vi "SP Append Group Data Fields.vi"(10 "S Parameter Results":T1={"Measurement Cycles"=0, "Sxx Data"=[], "S Parameter Test Parameters"={"Stimulus"={"Use Instrument Settings"=FALSE, "Blank Frequencies"=FALSE, "Sweep Type"=enum."Linear", "Sweep"={"Fstart"=500.0, "Fstop"=1500.0, "Units"=enum."MHz", "Points"=2}, "Power (dBm)"=999.0, "IFBW (Hz)"=-1.0, "Sweep Time (s)"=-1.0, "Calibration"={"State"=FALSE, "String"=""}}, "Measurement"={"Auto Select"=TRUE, "Data Source"=enum."VNA", "Ports"=2, "Parameters"=[]}, "De-Embed"={"De-Embed"=FALSE, "Adapters"=[]}, "Display"={"Lock Control"=FALSE, "Retain Settings"=TRUE, "Formatted Data"=FALSE, "Plot Orientation"=enum."Single", "Plot Controls"=[{"Trace Orientation"=enum."Overlay", "Frequency"={"Change Frequency"=FALSE, "Start"=500.0, "Stop"=1500.0, "Units"=enum."MHz"}, "Markers"=[], "Traces"=[]}, {"Trace Orientation"=enum."Overlay", "Frequency"={"Change Frequency"=FALSE, "Start"=500.0, "Stop"=1500.0, "Units"=enum."MHz"}, "Markers"=[], "Traces"=[]}, {"Trace Orientation"=enum."Overlay", "Frequency"={"Change Frequency"=FALSE, "Start"=500.0, "Stop"=1500.0, "Units"=enum."MHz"}, "Markers"=[], "Traces"=[]}, {"Trace Orientation"=enum."Overlay", "Frequency"={"Change Frequency"=FALSE, "Start"=500.0, "Stop"=1500.0, "Units"=enum."MHz"}, "Markers"=[], "Traces"=[]}]}, "Limits"=[], "Filter Limits"=[]}, "Instrument Used"={"ixInstrument"=0, "sxInstrumentId"="", "sDriverId"="", "sDriverType"="", "sSerialNumber"="", "tLastCalibration"=timestamp(0 s since 1904-01-01), "tCalibrationDue"=timestamp(0 s since 1904-01-01), "sConfiguration"=""}} {"S Parameter Test Parameters"."Filter Limits"."Parameter"."Stimulus Port" min=1 step=1; "S Parameter Test Parameters"."Filter Limits"."Parameter"."Response Port" min=1 step=1; "S Parameter Test Parameters"."Filter Limits"."Passband"."Bandwidth Attn" format="%.3g"; "S Parameter Test Parameters"."Filter Limits"."Passband"."Stop/Span" format="%.3g"; "S Parameter Test Parameters"."Filter Limits"."Passband"."Start/Center" format="%.3g"; "S Parameter Test Parameters"."Measurement"."Parameters"."Channel" min=0 max=32 step=1; "S Parameter Test Parameters"."Measurement"."Parameters"."Parameter"."Stimulus Port" min=1 step=1; "S Parameter Test Parameters"."Measurement"."Parameters"."Parameter"."Response Port" min=1 step=1; "S Parameter Test Parameters"."Limits"."Parameter"."Stimulus Port" min=1 step=1; "S Parameter Test Parameters"."Limits"."Parameter"."Response Port" min=1 step=1; "S Parameter Test Parameters"."Stimulus"."Sweep Time (s)" format="%.3g"; "S Parameter Test Parameters"."Display"."Plot Controls"."Traces"."Reference" format="%#.2g"; "S Parameter Test Parameters"."Display"."Plot Controls"."Traces"."Scale" min=0.001 step=1.0 format="%#.2g"; "S Parameter Test Parameters"."Display"."Plot Controls"."Traces"."Position" min=0.0 max=10.0; "S Parameter Test Parameters"."Display"."Plot Controls"."Frequency"."Stop" format="%.3g"; "S Parameter Test Parameters"."Display"."Plot Controls"."Frequency"."Start" format="%.3g"}, 11 "Fields In":T34[](array[typedef])) -> (3 "Fields Out":T34[](array[typedef]))   [LabVIEW 2011]
uses:
  server/database/Fields/Field Record.ctl
  server/database/Fields/Field DataTypes.ctl
  server/database/Fields/Field NextItem.ctl
  TypeDefs/SP Results.ctl
  TypeDefs/SP Test Parameters.ctl
  TypeDefs/SP Stimulus Parameters.ctl
  TypeDefs/SP Frequency Units.ctl
  TypeDefs/SP Calibration State.ctl
  TypeDefs/SP Measurement.ctl
  TypeDefs/SP Parameters.ctl
  TypeDefs/SP Parameter.ctl
  TypeDefs/SP De-Embed.ctl
  TypeDefs/SP Adapter.ctl
  TypeDefs/SP Data.ctl
  TypeDefs/SP Display Parameters.ctl
  TypeDefs/SP Display Plot Controls Cluster.ctl
  TypeDefs/SP Marker Cluster.ctl
  TypeDefs/SP Marker Type.ctl
  TypeDefs/SP Display Trace Controls.ctl
  TypeDefs/SP Display Format.ctl
  TypeDefs/SP Display Data.ctl
  TypeDefs/SP Limit.ctl
  TypeDefs/SP Format.ctl
  TypeDefs/SP Limit Type.ctl
  TypeDefs/SP Limit Point.ctl
  Test Referential Limit.ctl
  TypeDefs/SP Filter.ctl
  TypeDefs/SP Filter Type.ctl
  TypeDefs/SP Filter Passband.ctl
  TypeDefs/SP Frequency Format.ctl
  TypeDefs/SP Filter Ripple.ctl
  TypeDefs/SP Attenuation Point.ctl
  TypeDefs/SP Attenuation Type.ctl
  TypeDefs/SP Skirt Rejection Point.ctl
  TypeDefs/SP Relative Loss.ctl
  server/database/Stations/Instruments/Instrument Record.ctl
panel:
  # "Div"
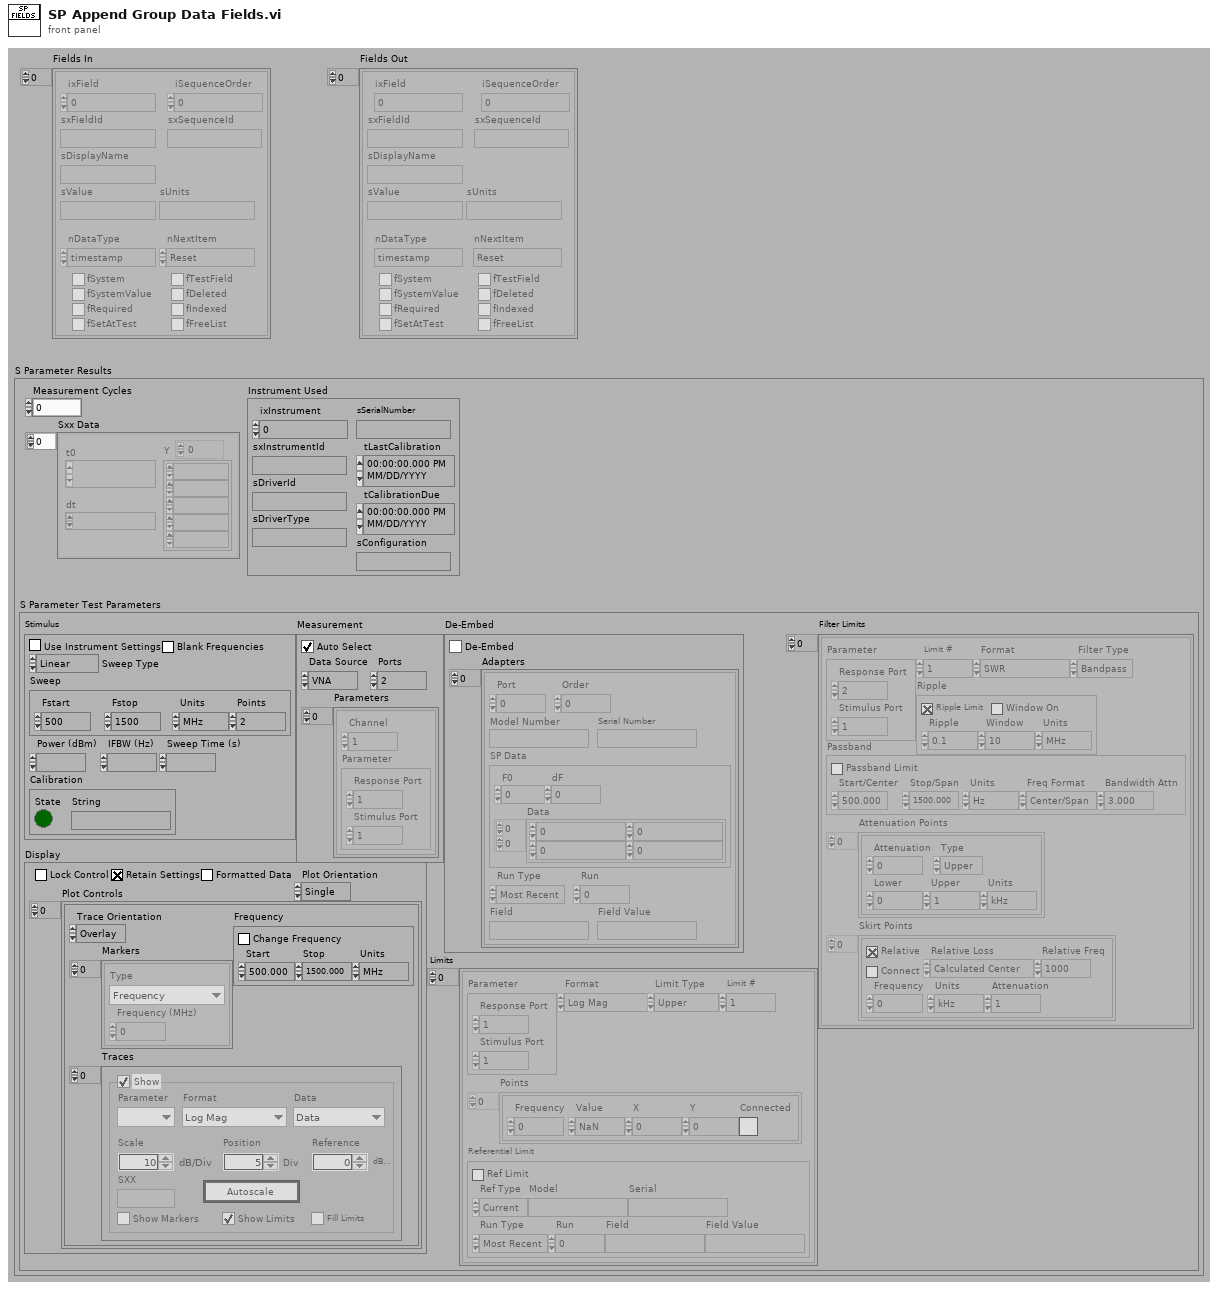
[diagram p1: front panel]
types:
  T1 = typedef "SP Results.ctl" = cluster{"Measurement Cycles":i32, "Sxx Data":waveform(dbl)[], "S Parameter Test Parameters":T2, "Instrument Used":T33}
  T2 = typedef "SP Test Parameters.ctl" = cluster{"Stimulus":T3, "Measurement":T6, "De-Embed":T9, "Display":T12, "Limits":T19[], "Filter Limits":T24[]}
  T3 = typedef "SP Stimulus Parameters.ctl" = cluster{"Use Instrument Settings":bool, "Blank Frequencies":bool, "Sweep Type":enum32{"Linear", "Logarithmic", "List", "Power", "CW"}, "Sweep":cluster{"Fstart":dbl, "Fstop":dbl, "Units":T4, "Points":i32}, "Power (dBm)":dbl, "IFBW (Hz)":dbl, "Sweep Time (s)":dbl, "Calibration":T5}
  T4 = typedef "SP Frequency Units.ctl" = enum16{"Hz", "kHz", "MHz", "GHz", "Points"}
  T5 = typedef "SP Calibration State.ctl" = cluster{"State":bool, "String":string}
  T6 = typedef "SP Measurement.ctl" = cluster{"Auto Select":bool, "Data Source":enum16{"VNA", "Data File"}, "Ports":i8, "Parameters":T7[]}
  T7 = typedef "SP Parameters.ctl" = cluster{"Channel":i8, "Parameter":T8}
  T8 = typedef "SP Parameter.ctl" = cluster{"Stimulus Port":i8, "Response Port":i8}
  T9 = typedef "SP De-Embed.ctl" = cluster{"De-Embed":bool, "Adapters":T10[]}
  T10 = typedef "SP Adapter.ctl" = cluster{"Port":i8, "Order":i8, "Model Number":string, "Serial Number":string, "SP Data":T11, "Run Type":enum16{"Most Recent", "Run #", "Match Field"}, "Run":i32, "Field":string, "Field Value":string}
  T11 = typedef "SP Data.ctl" = cluster{"F0":dbl, "dF":dbl, "Data":cdb[][]}
  T12 = typedef "SP Display Parameters.ctl" = cluster{"Lock Control":bool, "Retain Settings":bool, "Formatted Data":bool, "Plot Orientation":enum32{"Single", "Dual", "Quad"}, "Plot Controls":T13[]}
  T13 = typedef "SP Display Plot Controls Cluster.ctl" = cluster{"Trace Orientation":enum32{"Overlay", "Split"}, "Frequency":cluster{"Change Frequency":bool, "Start":dbl, "Stop":dbl, "Units":T4}, "Markers":T14[], "Traces":T16[]}
  T14 = typedef "SP Marker Cluster.ctl" = cluster{"Type":T15, "Frequency (MHz)":dbl}
  T15 = typedef "SP Marker Type.ctl" = enum16{"Frequency", "Trace Maximum", "Trace Minimum", "Limit Maximum", "Limit Minimum"}
  T16 = typedef "SP Display Trace Controls.ctl" = cluster{"Trace On":bool, "Measure":i32, "Format":T17, "Autoscale":bool, "Reference":dbl, "\nRefUnit":string, "Position":dbl, "Scale":dbl, "ScaleUnit":string, "LimitOn":bool, "LimitFill":bool, "Display Data":T18, "Show Markers":bool, "SXX":string}
  T17 = typedef "SP Display Format.ctl" = i32
  T18 = typedef "SP Display Data.ctl" = u16
  T19 = typedef "SP Limit.ctl" = cluster{"Parameter":T8, "Format":T20, "Limit Type":T21, "Points":T22[], "Referential Limit":T23, "Limit #":i8}
  T20 = typedef "SP Format.ctl" = enum16{"Log Mag", "Lin Mag", "SWR", "Phase", "Expanded Phase", "Delay", "Insertion Loss", "Isolation", "Return Loss"}
  T21 = typedef "SP Limit Type.ctl" = enum16{"Upper", "Lower", "Delta", "Filter", "Referential"}
  T22 = typedef "SP Limit Point.ctl" = cluster{"Frequency":dbl, "Value":dbl, "X":dbl, "Y":dbl, "Connected":bool}
  T23 = typedef "Test Referential Limit.ctl" = cluster{"Ref Limit":bool, "Ref Type":enum16{"Current", "Specify"}, "Model":string, "Serial":string, "Run Type":enum16{"Most Recent", "Run #", "Match Field"}, "Run":i32, "Field":string, "Field Value":string}
  T24 = typedef "SP Filter.ctl" = cluster{"Limit #":i8, "Parameter":T8, "Format":T20, "Filter Type":T25, "Passband":T26, "Ripple":T28, "Attenuation Points":T29[], "Skirt Points":T31[]}
  T25 = typedef "SP Filter Type.ctl" = enum16{"Lowpass", "Highpass", "Bandpass", "Bandstop"}
  T26 = typedef "SP Filter Passband.ctl" = cluster{"Start/Center":dbl, "Stop/Span":dbl, "Units":T4, "Freq Format":T27, "Bandwidth Attn":dbl, "Passband Limit":bool}
  T27 = typedef "SP Frequency Format.ctl" = enum16{"Start/Stop", "Center/Span"}
  T28 = typedef "SP Filter Ripple.ctl" = cluster{"Ripple Limit":bool, "Window On":bool, "Ripple":dbl, "Window":dbl, "Units":T4}
  T29 = typedef "SP Attenuation Point.ctl" = cluster{"Attenuation":dbl, "Type":T30, "Lower":dbl, "Upper":dbl, "Units":T4}
  T30 = typedef "SP Attenuation Type.ctl" = enum16{"Center", "Lower", "Upper"}
  T31 = typedef "SP Skirt Rejection Point.ctl" = cluster{"Relative":bool, "Connect":bool, "Frequency":dbl, "Units":T4, "Attenuation":dbl, "Relative Loss":T32, "Relative Freq":dbl}
  T32 = typedef "SP Relative Loss.ctl" = enum16{"Calculated Center", "Passband Minimum", "Passband Maximum", "Passband Average", "Frequency"}
  T33 = typedef "Instrument Record.ctl" = cluster{"ixInstrument":i32, "sxInstrumentId":string, "sDriverId":string, "sDriverType":string, "sSerialNumber":string, "tLastCalibration":timestamp, "tCalibrationDue":timestamp, "sConfiguration":string}
  T34 = typedef "Field Record.ctl" = cluster{"ixField":i32, "iSequenceOrder":i32, "sxFieldId":string, "sxSequenceId":string, "sDisplayName":string, "sValue":string, "sUnits":string, "nDataType":T35, "nNextItem":T36, "fSystem":bool, "fSystemValue":bool, "fRequired":bool, "fSetAtTest":bool, "fTestField":bool, "fDeleted":bool, "fIndexed":bool, "fFreeList":bool}
  T35 = typedef "Field DataTypes.ctl" = enum32{"text", "numeric", "list", "timestamp", "boolean"}
  T36 = typedef "Field NextItem.ctl" = enum32{"Reset", "Retain", "Auto-Increment"}
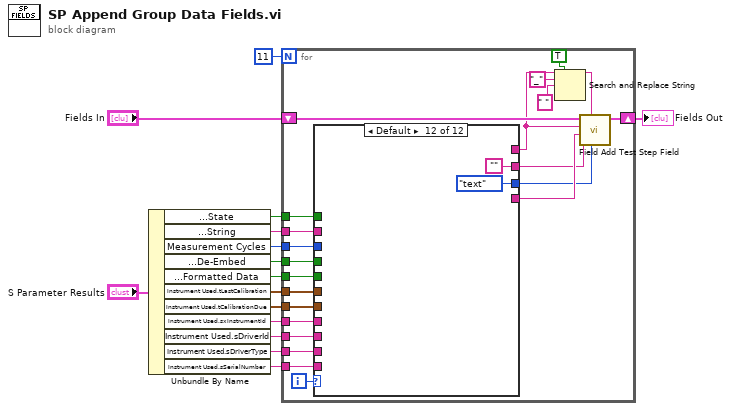
[diagram p0: block diagram]
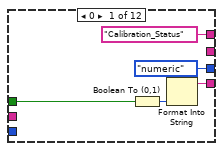
[diagram p2: hidden frame]
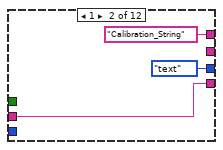
[diagram p3: hidden frame]
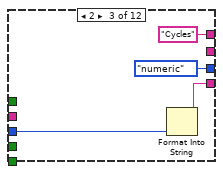
[diagram p4: hidden frame]
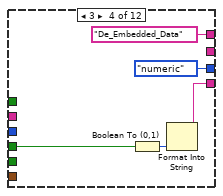
[diagram p5: hidden frame]
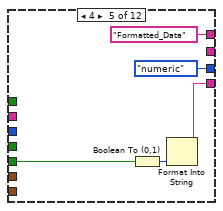
[diagram p6: hidden frame]
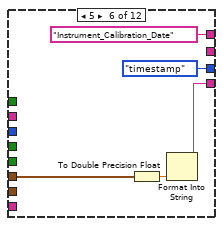
[diagram p7: hidden frame]
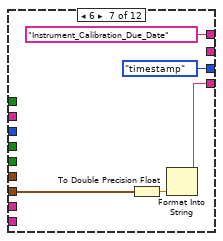
[diagram p8: hidden frame]
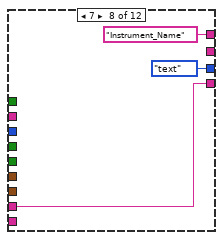
[diagram p9: hidden frame]
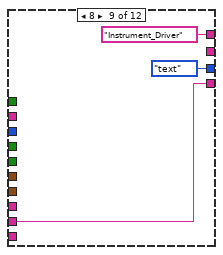
[diagram p10: hidden frame]
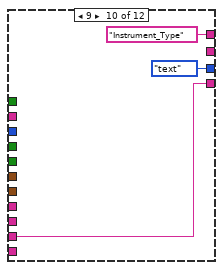
[diagram p11: hidden frame]
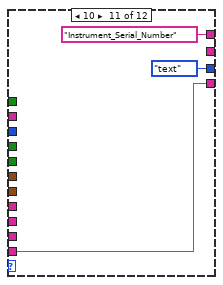
[diagram p12: hidden frame]
diagram:
  n1 = Unbundle By Name("S Parameter Results") -> ("S Parameter Test Parameters.Stimulus.Calibration.State"=w11:bool, "S Parameter Test Parameters.Stimulus.Calibration.String"=w10:string, "Measurement Cycles"=w9:i32, "S Parameter Test Parameters.De-Embed.De-Embed"=w8:bool, "S Parameter Test Parameters.Display.Formatted Data"=w7:bool, "Instrument Used.tLastCalibration"=w6:timestamp, "Instrument Used.tCalibrationDue"=w5:timestamp, "Instrument Used.sxInstrumentId"=w4:string, "Instrument Used.sDriverId"=w3:string, "Instrument Used.sDriverType"=w2:string, "Instrument Used.sSerialNumber"=w1:string)
  n2 = for {
    N: 11 -> [_]
    tunnel: w7 -> [w36]
    tunnel: w8 -> [w35]
    tunnel: w9 -> [w34]
    tunnel: w10 -> [w33]
    tunnel: w11 -> [w32]
    shift-right: [w30] -> w14
    shift-left: "Fields In" -> [w31]
    tunnel: w6 -> [w26]
    tunnel: w5 -> [w25]
    tunnel: w4 -> [w24]
    tunnel: w3 -> [w23]
    tunnel: w2 -> [w22]
    tunnel: w1 -> [w21]
    i -> [w37]
    n3 = case shown="Default" w37 {
      tunnel: w36 -> [_ _ _ _ w56 _ _ _ _ _ _ _]
      tunnel: w35 -> [_ _ _ w51 _ _ _ _ _ _ _ _]
      tunnel: w34 -> [_ _ w47 _ _ _ _ _ _ _ _ _]
      tunnel: w33 -> [_ w43 _ _ _ _ _ _ _ _ _ _]
      tunnel: w32 -> [w39 _ _ _ _ _ _ _ _ _ _ _]
      tunnel: ["Calibration_Status" ("Field_ID") "Calibration_String" ("Field_ID") "Cycles" ("Field_ID") "De_Embedded_Data" ("Field_ID") "Formatted_Data" ("Field_ID") "Instrument_Calibration_Date" ("Field_ID") "Instrument_Calibration_Due_Date" ("Field_ID") "Instrument_Name" ("Field_ID") "Instrument_Driver" ("Field_ID") "Instrument_Type" ("Field_ID") "Instrument_Serial_Number" ("Field_ID") _] -> w16
      tunnel: [Field_DataTypes."numeric" ("Data Type") Field_DataTypes."text" ("Data Type") Field_DataTypes."numeric" ("Data Type") Field_DataTypes."numeric" ("Data Type") Field_DataTypes."numeric" ("Data Type") Field_DataTypes."timestamp" ("Data Type") Field_DataTypes."timestamp" ("Data Type") Field_DataTypes."text" ("Data Type") Field_DataTypes."text" ("Data Type") Field_DataTypes."text" ("Data Type") Field_DataTypes."text" ("Data Type") Field_DataTypes."text" ("Data Type")] -> w28
      tunnel: [w41 w43 w46 w50 w58 w63 w68 w70 w73 w76 w79 _] -> w29
      tunnel: [_ _ _ _ _ _ _ _ _ _ _ ""] -> w27
      tunnel: w26 -> [_ _ _ _ _ w60 _ _ _ _ _ _]
      tunnel: w25 -> [_ _ _ _ _ _ w65 _ _ _ _ _]
      tunnel: w24 -> [_ _ _ _ _ _ _ w70 _ _ _ _]
      tunnel: w23 -> [_ _ _ _ _ _ _ _ w73 _ _ _]
      tunnel: w22 -> [_ _ _ _ _ _ _ _ _ w76 _ _]
      tunnel: w21 -> [_ _ _ _ _ _ _ _ _ _ w79 _]
      frame 0 {
        n4 = Boolean To (0,1)(Boolean=w39) -> (0, 1=w38:i16)
        n5 = Format Into String(w38) -> (resulting string=w41:string)  [unwired: 3 in, 1 out]
      }
      frame 1 {
      }
      frame 2 {
        n6 = Format Into String(w47) -> (resulting string=w46:string)  [unwired: 3 in, 1 out]
      }
      frame 3 {
        n7 = Boolean To (0,1)(Boolean=w51) -> (0, 1=w52:i16)
        n8 = Format Into String(w52) -> (resulting string=w50:string)  [unwired: 3 in, 1 out]
      }
      frame 4 {
        n9 = Boolean To (0,1)(Boolean=w56) -> (0, 1=w55:i16)
        n10 = Format Into String(w55) -> (resulting string=w58:string)  [unwired: 3 in, 1 out]
      }
      frame 5 {
        n11 = To Double Precision Float(number=w60) -> (double precision float=w61:dbl)
        n12 = Format Into String(w61) -> (resulting string=w63:string)  [unwired: 3 in, 1 out]
      }
      frame 6 {
        n13 = To Double Precision Float(number=w65) -> (double precision float=w66:dbl)
        n14 = Format Into String(w66) -> (resulting string=w68:string)  [unwired: 3 in, 1 out]
      }
      frame 7 {
      }
      frame 8 {
      }
      frame 9 {
      }
      frame 10 {
      }
      frame Default {
      }
    }
    n15 = Search and Replace String(replace all?=TRUE ("replace all? (F)"), input string=w16, search string="_", replace string=" " ("replace string (\"\")")) -> (result string=w17:string)  [unwired: 1 in, 6 out]
    n16 = call "Field Add Test Step Field.vi"("nDataType"=w28, "sDisplayName"=w17, "sUnits"=w27, "sValue"=w29, "sxFieldId"=w16, "Fields In"=w31) -> ("Fields Out"=w30:T34[])  [unwired: 5 out]
  }
  "Fields Out" <- w14
